vi "DAC Configure.vi"(8 "error in":errorcluster, 11 "DAC ADV in":refnum<class "DAC ADV.lvclass">) -> (0 "error out":errorcluster, 3 "DAC ADV out":refnum<class "DAC ADV.lvclass">)   [LabVIEW 2019, in "DAC.lvlib" / "DAC ADV.lvclass"]
uses:
  DAC ADV.lvclass
  C:/Users/krio/Documents/LV_Projects/test-stand/App/DAC/DAC.lvclass
  DAC.lvclass/DAC.ctl
  DAC ADV.lvclass/DAC ADV.ctl
  <vilib>/DAQmx/create/channels.llb/DAQmx Create Channel (AI-Voltage-Basic).vi
  DAC.lvclass
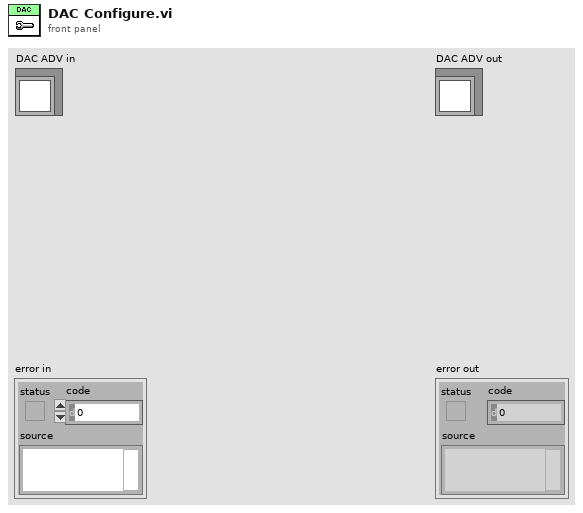
[diagram p1: front panel]
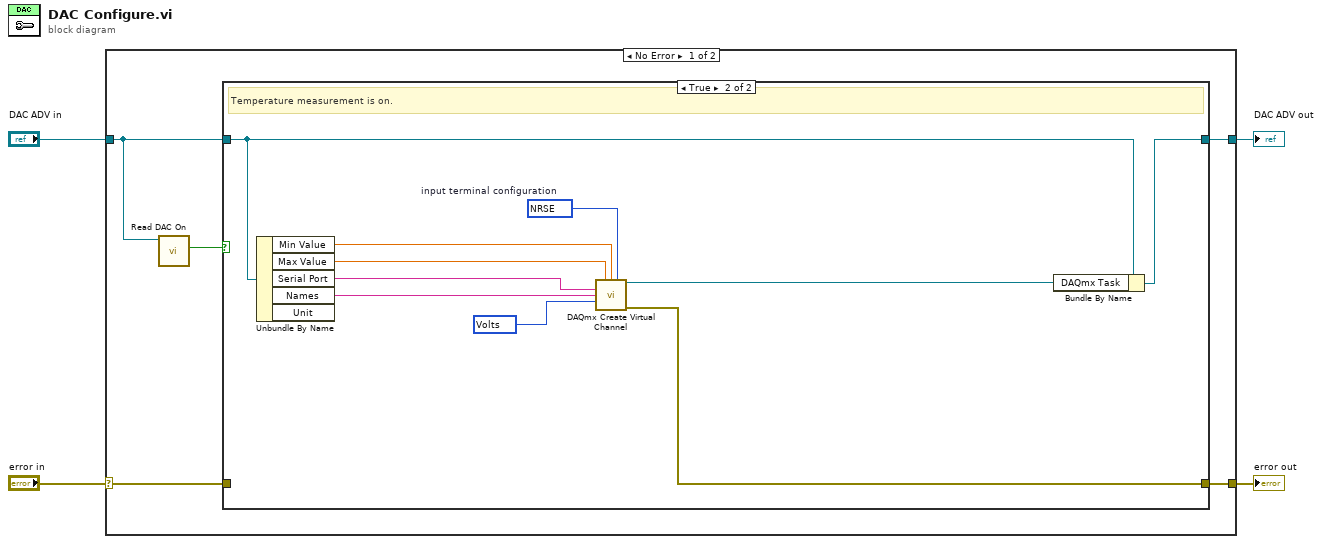
[diagram p0: block diagram]
diagram:
  n1 = case shown="No Error" "error in" {
    selector: "error in" -> [w6 w23]
    tunnel: [w5 w23] -> w4
    tunnel: [w7 w22] -> w3
    tunnel: "DAC ADV in" -> [w9 w22]
    frame No Error {
      n2 = call "Read DAC On.vi"("DAC in"=w9) -> ("DAC On"=w8:bool)  [unwired: 8 in, 2 out]
      n3 = case shown="True" w8 {
        tunnel: w9 -> [w11 w19]
        tunnel: [w11 w18] -> w7
        tunnel: w6 -> [w10 _]
        tunnel: [w10 w17] -> w5
        frame False {
          # "Temperature measurement is off."
        }
        frame True {
          w12 = 10078 items=["Default"=-1, "RSE"=10083, "NRSE"=10078, "Differential"=10106, "Pseudodifferential"=12529]  # input terminal configuration
          w13 = 10348 items=["Volts"=10348, "From Custom Scale"=10065] ("units")
          # "Temperature measurement is on."
          n4 = Unbundle By Name(w19) -> ("Min Value"=w20:dbl, "Max Value"=w21:dbl, "Serial Port"=w16:string, "Names"=w15:string)  [unwired: 1 out]
          n5 = call-poly <vilib>:"DAQmx Create Virtual Channel.vi"("maximum value"=w21, "minimum value"=w20, "input terminal configuration"=w12, "physical channels"=w16, "name to assign"=w15, "units"=w13) -> ("task out"=w14:refnum<k21>, "error out"=w17:errorcluster)  [unwired: 8 in]
          n6 = Bundle By Name(cluster=w19, "DAQmx Task"=w14) -> (w18:refnum<class "DAC ADV.lvclass">)
        }
      }
    }
    frame Error {
    }
  }
  "error out" <- w4
  "DAC ADV out" <- w3
